vi "CleanHandler_Contents.vi"   [LabVIEW 2014, in "CleanHandler.lvlib"]
uses:
  CleanHandler.lvlib
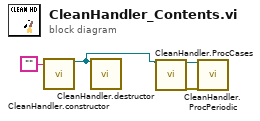
[diagram p0: block diagram]
diagram:
  n1 = call "CleanHandler.constructor.vi"("name"="") -> ("i ref out"=w1:refnum<vi>)  [unwired: 16 in, 2 out]
  n2 = call "CleanHandler.destructor.vi"("i ref in"=w1) -> ()  [unwired: 18 in, 1 out]
  n3 = call "CleanHandler.ProcCases.vi"("i ref in"=w1) -> ("i ref out"=w3:refnum<vi>, "error out"=w2:errorcluster)  [unwired: 16 in, 1 out]
  n4 = call "CleanHandler.ProcPeriodic.vi"("i ref in"=w3, "error in (no error)"=w2) -> ()  [unwired: 15 in, 3 out]
